vi "VIs Folder Path.vi"(8 "error in (no error)":errorcluster, 9 "Operation":enum16{"Get", "Set"}(ring), 11 "Path":path) -> (0 "error out":errorcluster, 3 "Path 2":path)   [LabVIEW 2020, in "WebServiceImporter.lvlib" / "VI Generator.lvlib"]
uses:
  <vilib>/Platform/WebService/VI Generator/VI Generator.lvlib
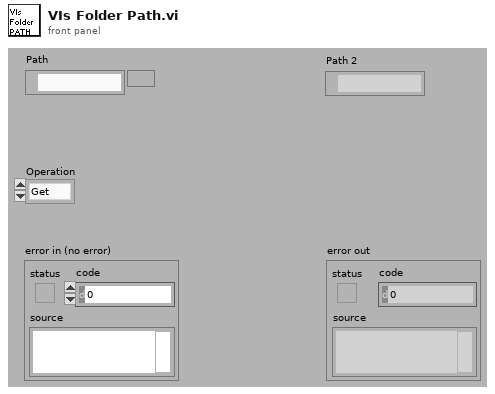
[diagram p1: front panel]
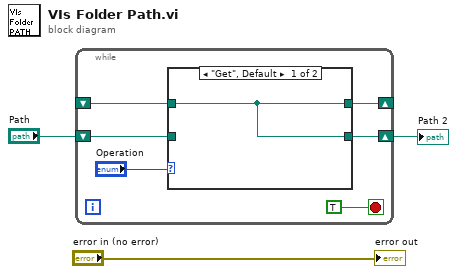
[diagram p0: block diagram]
diagram:
  n1 = while {
    shift-right: [w6] -> w1
    shift-left: "Path" -> [w7]
    shift-right: [w5] -> _
    shift-left: _ -> [w4]
    stop <- TRUE stop-if-true
    n2 = case shown="\"Get\", Default" "Operation" {
      tunnel: w7 -> [_ w11]
      tunnel: [w10 w11] -> w6
      tunnel: [w10 w11] -> w5
      tunnel: w4 -> [w10 _]
      frame "Get", Default {
      }
      frame "Set" {
      }
    }
  }
  "Path 2" <- w1
  "error out" <- "error in (no error)"
